vi "Update Exposure Time.vi"(8 "error in (no error)":errorcluster, 10 "Value":string, 11 "Bobcat 640 in":refnum<class "Bobcat 640.lvclass">) -> (0 "error out":errorcluster, 3 "Bobcat 640 out":refnum<class "Bobcat 640.lvclass">)   [LabVIEW 2018, in "Bobcat 640.lvlib" / "Bobcat 640.lvclass"]
uses:
  Bobcat 640.lvclass
  Bobcat 640.lvclass/Bobcat 640.ctl
  <resource>/objmgr/imaqdx.rc
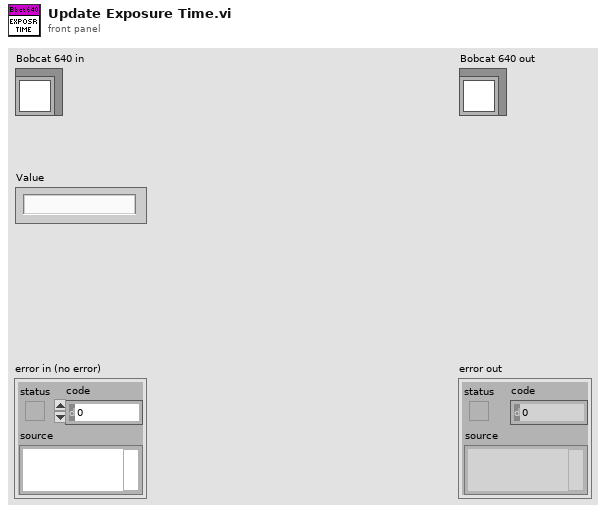
[diagram p1: front panel]
types:
  T1 = typedef "IMAQdx.ctl" = refnum<k21>
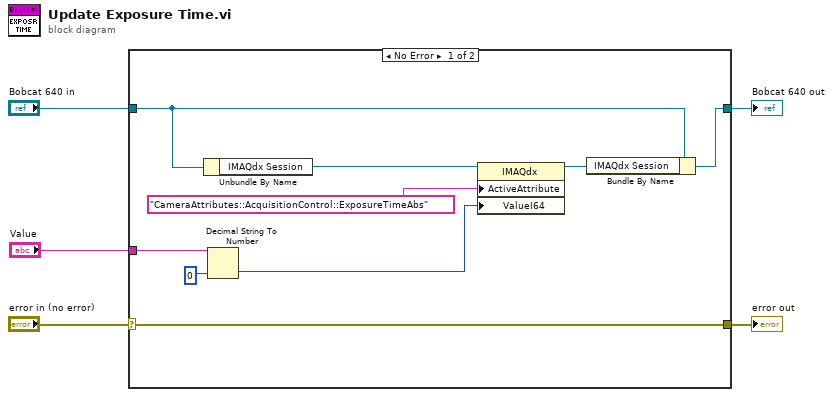
[diagram p0: block diagram]
diagram:
  n1 = case shown="No Error" "error in (no error)" {
    selector: "error in (no error)" -> [w14 w16]
    tunnel: [w14 w16] -> w4
    tunnel: [w6 w15] -> w2
    tunnel: "Bobcat 640 in" -> [w8 w15]
    tunnel: "Value" -> [w12 _]
    frame No Error {
      n2 = Unbundle By Name(w8) -> ("IMAQdx Session"=w9:T1)
      n3 = Decimal String To Number(string=w12, default (0L)=i64 0 ("ValueI64")) -> (number=w10:i64)  [unwired: 1 in, 1 out]
      n4 = property class="IMAQdx"(reference=w9, "ActiveAttribute"="CameraAttributes::AcquisitionControl::ExposureTimeAbs", "ValueI64"=w10) -> (reference out=w7:T1)  [unwired: 1 in, 1 out]
      n5 = Bundle By Name(cluster=w8, "IMAQdx Session"=w7) -> (w6:refnum<class "Bobcat 640.lvclass">)
    }
    frame Error {
    }
  }
  "error out" <- w4
  "Bobcat 640 out" <- w2
